vi "6000_watchdog_configure.vi"() -> ()   [LabVIEW 2010]
panel:
  in  "Port Name":string="MainNetwork"
  in  "Array":bool[](array[boolean])
  in  "100ms Intervals":u8
  in  "Host Watchdog":bool
  out "Reply":string
  in  "Module Address":u8
  # "0    1   2    3"
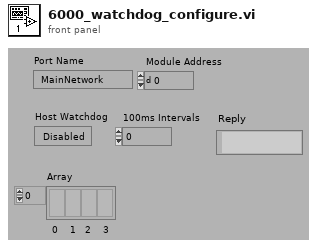
[diagram p1: front panel]
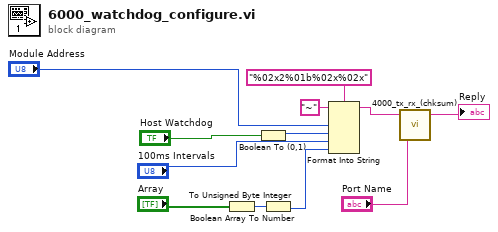
[diagram p0: block diagram]
diagram:
  n1 = Boolean Array To Number(Boolean array="Array") -> (number=w11:u32)
  n2 = Boolean To (0,1)(Boolean="Host Watchdog") -> (0, 1=w9:i16)
  n3 = To Unsigned Byte Integer(number=w11) -> (unsigned 8bit integer=w4:u8)
  n4 = Format Into String(format string="%02x2%01b%02x%02x" ("Format String"), initial string="~" ("Input String"), "Module Address", w9, "100ms Intervals", w4) -> (resulting string=w3:string)  [unwired: 1 in, 1 out]
  n5 = call "4000_tx_rx_(chksum).vi"("Port Name"="Port Name", "Write String"=w3) -> ("Read"=→"Reply":string)  [unwired: 1 in, 2 out]
